vi "ContinueDoingQnsPaper1(SubVI).vi"(8 "RefPrevious":refnum<vi>, 9 "RefNext":refnum<vi>, 11 "connection reference":T1) -> ()   [LabVIEW 2013]
uses:
  <vilib>/addons/database/Connection.llb/Conn ObjectReference.ctl
  FYP_LabviewGlobal(SubVI).vi
  <vilib>/addons/database/_DB Variant To Data/Database Variant To Data.xnode
  <vilib>/addons/database/NI_Database_API.lvlib
panel:
  out "Choice":string
  out "D":bool
  out "C":bool
  out "B":bool
  out "A":bool
  out "D":string
  out "C":string
  out "B":string
  out "A":string
  out "Question":string
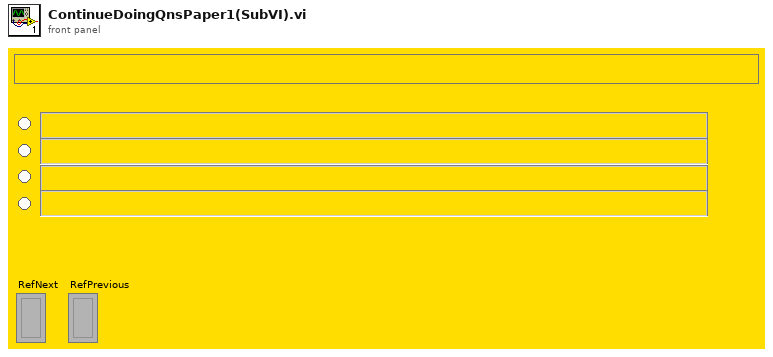
[diagram p1: front panel]
types:
  T1 = typedef "NI_Database_API.lvlib/Conn ObjectReference.ctl" = refnum<k1>
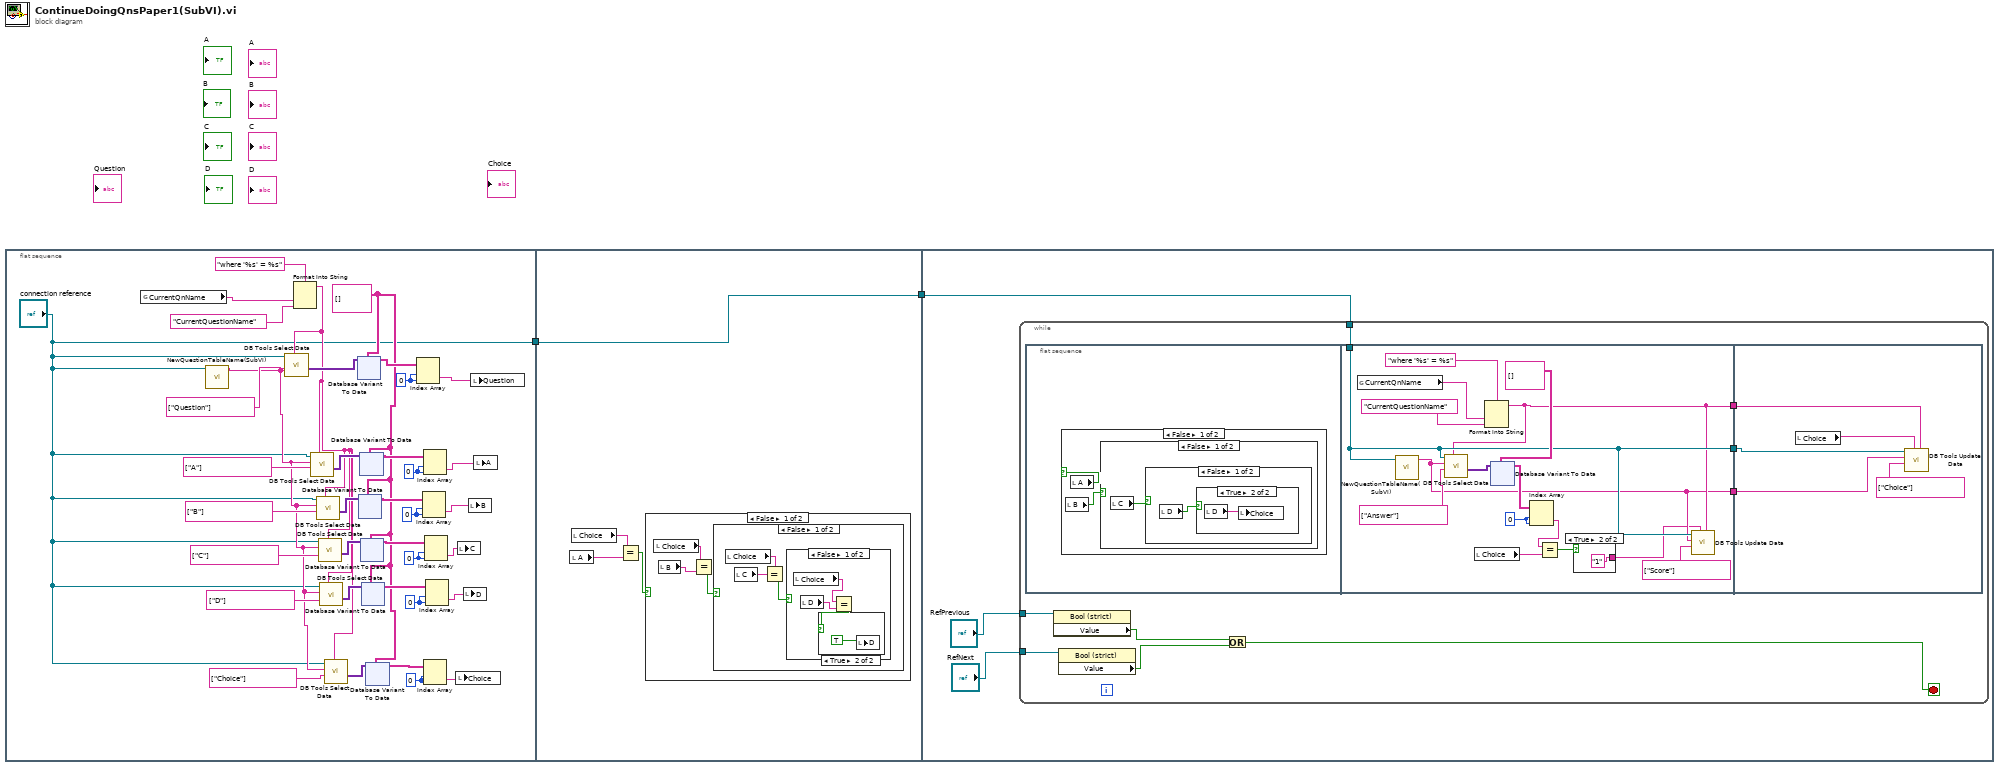
[diagram p0: block diagram]
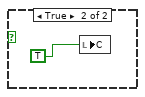
[diagram p3: hidden frame]
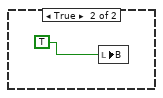
[diagram p4: hidden frame]
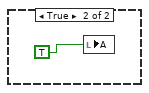
[diagram p5: hidden frame]
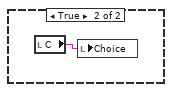
[diagram p7: hidden frame]
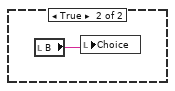
[diagram p8: hidden frame]
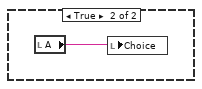
[diagram p9: hidden frame]
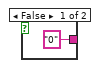
[diagram p10: hidden frame]
diagram:
  n1 = flat-sequence {
    tunnel: ["connection reference"] -> w1
    tunnel: [w304] -> w2
    tunnel: w1 -> [w304]
    tunnel: w2 -> [w323]
    frame #0 {
      w14 = 0 ("disabled index (col)")
      w19 = 0 ("disabled index (col)")
      w24 = 0 ("disabled index (col)")
      w28 = 0 ("disabled index (col)")
      w32 = 0 ("disabled index (col)")
      w35 = 0 ("disabled index (col)")
      w11 = string[][] []
      n2 = global read "FYP_LabviewGlobal(SubVI).vi" "CurrentQnName"() -> (w3:string)
      n3 = call "NewQuestionTableName(SubVI).vi"("connection reference"="connection reference") -> ("String"=w8:string)  [unwired: 9 in, 1 out]
      n4 = Format Into String(format string="where '%s' = %s", w3, "CurrentQuestionName") -> (resulting string=w5:string)  [unwired: 2 in, 1 out]
      n5 = call <vilib>:"DB Tools Select Data.vi"("condition"=w5, "columns"=string[] ["Question"], "table"=w8, "connection reference"="connection reference") -> ("data"=w38:variant[][])  [unwired: 2 in, 2 out]
      n6 = call <vilib>:"DB Tools Select Data.vi"("condition"=w5, "columns"=string[] ["A"], "table"=w8, "connection reference"="connection reference") -> ("data"=w33:variant[][])  [unwired: 2 in, 2 out]
      n7 = call <vilib>:"DB Tools Select Data.vi"("condition"=w5, "columns"=string[] ["B"], "table"=w8, "connection reference"="connection reference") -> ("data"=w26:variant[][])  [unwired: 2 in, 2 out]
      n8 = call <vilib>:"DB Tools Select Data.vi"("condition"=w5, "columns"=string[] ["C"], "table"=w8, "connection reference"="connection reference") -> ("data"=w22:variant[][])  [unwired: 2 in, 2 out]
      n9 = call <vilib>:"DB Tools Select Data.vi"("condition"=w5, "columns"=string[] ["D"], "table"=w8, "connection reference"="connection reference") -> ("data"=w17:variant[][])  [unwired: 2 in, 2 out]
      n10 = call <vilib>:"DB Tools Select Data.vi"("condition"=w5, "columns"=string[] ["Choice"], "table"=w8, "connection reference"="connection reference") -> ("data"=w12:variant[][])  [unwired: 2 in, 2 out]
      n11 = xnode "Database Variant To Data"("database variant"=w38, "type"=w11) -> ("data"=w37:string[][])  [unwired: 1 in, 1 out]
      n12 = xnode "Database Variant To Data"("database variant"=w26, "type"=w11) -> ("data"=w27:string[][])  [unwired: 1 in, 1 out]
      n13 = xnode "Database Variant To Data"("database variant"=w33, "type"=w11) -> ("data"=w31:string[][])  [unwired: 1 in, 1 out]
      n14 = xnode "Database Variant To Data"("database variant"=w22, "type"=w11) -> ("data"=w23:string[][])  [unwired: 1 in, 1 out]
      n15 = xnode "Database Variant To Data"("database variant"=w17, "type"=w11) -> ("data"=w18:string[][])  [unwired: 1 in, 1 out]
      n16 = xnode "Database Variant To Data"("database variant"=w12, "type"=w11) -> ("data"=w13:string[][])  [unwired: 1 in, 1 out]
      n17 = Index Array(array=w37, index (row)=w35, index (col)=w35) -> (element=w36:string)
      n18 = Index Array(array=w27, index (row)=w28, index (col)=w28) -> (element=w25:string)
      n19 = Index Array(array=w31, index (row)=w32, index (col)=w32) -> (element=w30:string)
      n20 = Index Array(array=w13, index (row)=w14, index (col)=w14) -> (element=w9:string)
      n21 = Index Array(array=w23, index (row)=w24, index (col)=w24) -> (element=w21:string)
      n22 = Index Array(array=w18, index (row)=w19, index (col)=w19) -> (element=w15:string)
      n23 = local write "Choice"(w9) -> ()
      n24 = local write "C"(w21) -> ()
      n25 = local write "D"(w15) -> ()
      n26 = local write "B"(w25) -> ()
      n27 = local write "Question"(w36) -> ()
      n28 = local write "A"(w30) -> ()
    }
    frame #1 {
      n29 = local read "A"() -> (w306:string)
      n30 = local read "Choice"() -> (w307:string)
      n31 = Equal?(x=w307, y=w306) -> (x = y?=w305:bool)
      n32 = case shown="False" w305 {
        frame False {
          n33 = local read "Choice"() -> (w310:string)
          n34 = local read "B"() -> (w309:string)
          n35 = Equal?(x=w310, y=w309) -> (x = y?=w308:bool)
          n36 = case shown="False" w308 {
            frame False {
              n37 = local read "Choice"() -> (w313:string)
              n38 = local read "C"() -> (w312:string)
              n39 = Equal?(x=w313, y=w312) -> (x = y?=w311:bool)
              n40 = case shown="False" w311 {
                frame False {
                  n41 = local read "Choice"() -> (w316:string)
                  n42 = local read "D"() -> (w315:string)
                  n43 = Equal?(x=w316, y=w315) -> (x = y?=w314:bool)
                  n44 = case shown="True" w314 {
                    frame False {
                    }
                    frame True {
                      n45 = local write "D"(TRUE) -> ()
                    }
                  }
                }
                frame True {
                  n46 = local write "C"(TRUE) -> ()
                }
              }
            }
            frame True {
              n47 = local write "B"(TRUE) -> ()
            }
          }
        }
        frame True {
          n48 = local write "A"(TRUE) -> ()
        }
      }
    }
    frame #2 {
      n49 = while {
        tunnel: w323 -> [w332]
        tunnel: "RefPrevious" -> [w328]
        tunnel: "RefNext" -> [w327]
        stop <- w324 stop-if-true
        n50 = flat-sequence {
          tunnel: w332 -> [w349]
          tunnel: [w349] -> w331
          tunnel: [w346] -> w330
          tunnel: [w348] -> w329
          tunnel: w331 -> [w406]
          tunnel: w330 -> [w405]
          tunnel: w329 -> [w404]
          frame #0 {
            n51 = local read "A"() -> (w333:bool)
            n52 = case shown="False" w333 {
              frame False {
                n53 = local read "B"() -> (w334:bool)
                n54 = case shown="False" w334 {
                  frame False {
                    n55 = local read "C"() -> (w335:bool)
                    n56 = case shown="False" w335 {
                      frame False {
                        n57 = local read "D"() -> (w336:bool)
                        n58 = case shown="True" w336 {
                          frame False {
                          }
                          frame True {
                            n59 = local read "D"() -> (w337:string)
                            n60 = local write "Choice"(w337) -> ()
                          }
                        }
                      }
                      frame True {
                        n61 = local read "C"() -> (w338:string)
                        n62 = local write "Choice"(w338) -> ()
                      }
                    }
                  }
                  frame True {
                    n63 = local read "B"() -> (w339:string)
                    n64 = local write "Choice"(w339) -> ()
                  }
                }
              }
              frame True {
                n65 = local read "A"() -> (w340:string)
                n66 = local write "Choice"(w340) -> ()
              }
            }
          }
          frame #1 {
            w350 = 0 ("disabled index (col)")
            n67 = global read "FYP_LabviewGlobal(SubVI).vi" "CurrentQnName"() -> (w341:string)
            n68 = call "NewQuestionTableName(SubVI).vi"("connection reference"=w349) -> ("String"=w346:string)  [unwired: 9 in, 1 out]
            n69 = local read "Choice"() -> (w344:string)
            n70 = Format Into String(format string="where '%s' = %s", w341, "CurrentQuestionName") -> (resulting string=w348:string)  [unwired: 2 in, 1 out]
            n71 = call <vilib>:"DB Tools Select Data.vi"("condition"=w348, "columns"=string[] ["Answer"], "table"=w346, "connection reference"=w349) -> ("data"=w353:variant[][])  [unwired: 2 in, 2 out]
            n72 = xnode "Database Variant To Data"("database variant"=w353, "type"=string[][] []) -> ("data"=w351:string[][])  [unwired: 1 in, 1 out]
            n73 = Index Array(array=w351, index (row)=w350, index (col)=w350) -> (element=w345:string)
            n74 = Equal?(x=w345, y=w344) -> (x = y?=w343:bool)
            n75 = case shown="True" w343 {
              tunnel: ["0" "1"] -> w342
              frame False {
              }
              frame True {
              }
            }
            n76 = call <vilib>:"DB Tools Update Data.vi"("condition"=w348, "data"=w342, "columns"=string[] ["Score"], "table"=w346, "connection reference"=w349) -> ()  [unwired: 5 in, 2 out]
          }
          frame #2 {
            n77 = local read "Choice"() -> (w403:string)
            n78 = call <vilib>:"DB Tools Update Data.vi"("condition"=w404, "data"=w403, "columns"=string[] ["Choice"], "table"=w405, "connection reference"=w406) -> ()  [unwired: 5 in, 2 out]
          }
        }
        n79 = property class="Bool (strict)"(reference=w328) -> ("Value"=w326:bool)  [unwired: 1 in, 2 out]
        n80 = property class="Bool (strict)"(reference=w327) -> ("Value"=w325:bool)  [unwired: 1 in, 2 out]
        n81 = Or(x=w326, y=w325) -> (x .or. y?=w324:bool)
      }
    }
  }
